vi "读取型号检测项.vi"(0 "产品型号路径":path, 5 "产品型号":string="potteryTemplete", 7 "树形List":refnum<vi>, 11 "error in (no error)":errorcluster caption="错误输入（无错误）") -> (15 "error out":errorcluster caption="错误输出")   [LabVIEW 2017]
uses:
  <vilib>/Utility/file.llb/Read Delimited Spreadsheet (string).vi
panel:
  out "添加的数组":string[][](array[string])
  out "大小":i32
  out "缩进格式数":i32[](array[numeric])
  out "all rows":string[][](array[string]) caption="所有行"
  out "添加的路径 2":path
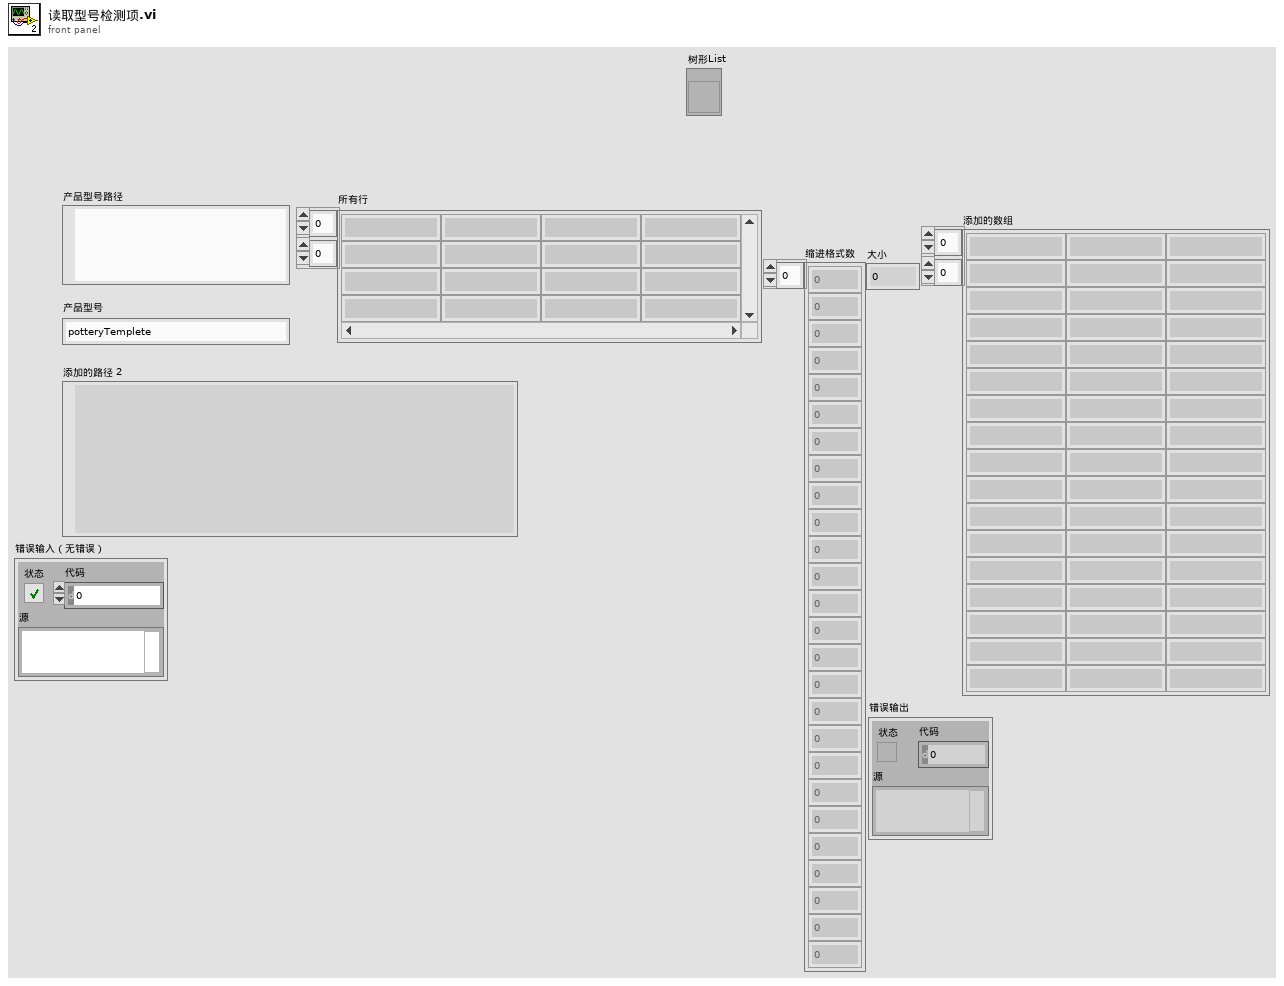
[diagram p1: front panel]
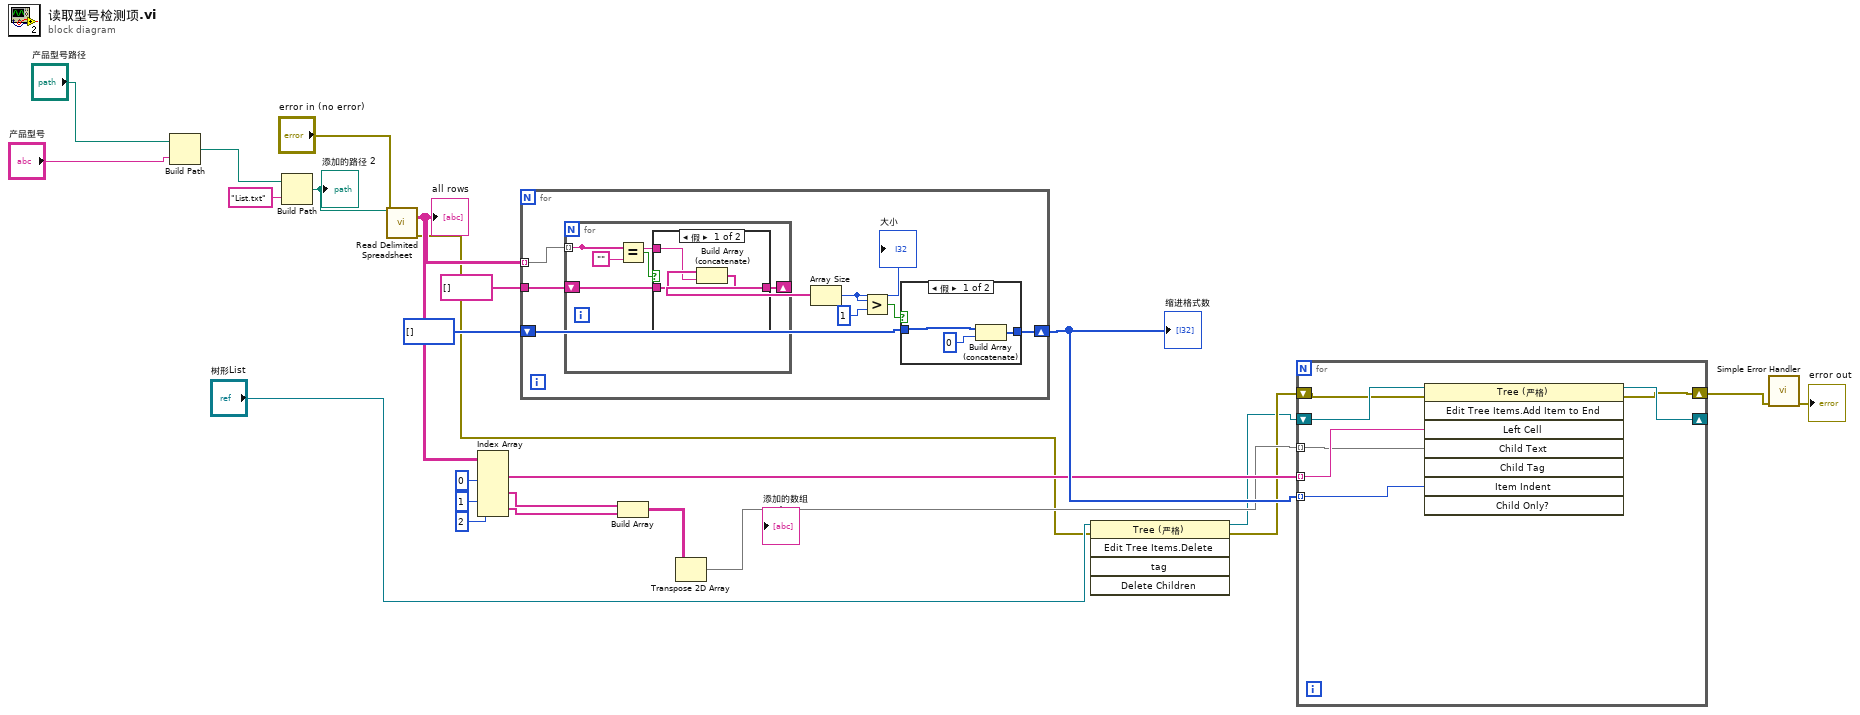
[diagram p0: block diagram]
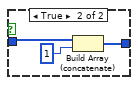
[diagram p3: hidden frame]
diagram:
  n1 = Build Path(base path="产品型号路径", name or relative path="产品型号") -> (appended path=w22:path)
  n2 = Build Path(base path=w22, name or relative path="List.txt" ("名称或相对路径")) -> (appended path=w20:path)
  "添加的路径 2" <- w20
  n3 = call-poly <vilib>:"Read Delimited Spreadsheet.vi"("file path (dialog if empty)"=w20, "error in (no error)"="error in (no error)") -> ("all rows"=w16:string[][], "error out"=w3:errorcluster)  [unwired: 8 in, 4 out]
  "all rows" <- w16
  n4 = Index Array(array=w16, index (col) #1=0 ("禁用的索引 (列)"), index (col) #2=1 ("索引 (列)"), index (col) #3=2 ("索引 (列)")) -> (element #1=w14:string[], element #2=w11:string[], element #3=w10:string[])  [unwired: 3 in]
  n5 = for {
    tunnel: w16 -> [w27] mode=indexing
    shift-right: [w28] -> w17
    shift-left: i32[] [] -> [w29]
    tunnel: string[] [] -> [w26]
    n6 = for {
      tunnel: w27 -> [w33] mode=indexing
      shift-right: [w34] -> w25
      shift-left: w26 -> [w35]
      n7 = Equal?(x=w33, y="") -> (x = y?=w36:bool)
      n8 = case shown="假" w36 {
        tunnel: w35 -> [w40 w41]
        tunnel: [w38 w41] -> w34
        tunnel: w33 -> [w39 _]
        frame False {
          n9 = Build Array (concatenate)(w40, w39) -> (w38:string[])
        }
        frame True {
        }
      }
    }
    n10 = Array Size(array=w25) -> (size(s)=w32:i32)
    "大小" <- w32
    n11 = Greater?(x=w32, y=1) -> (0:w30:bool)
    n12 = case shown="假" w30 {
      tunnel: w29 -> [w43 w47]
      tunnel: [w42 w45] -> w28
      frame False {
        n13 = Build Array (concatenate)(w43, 0 ("y")) -> (w42:i32[])
      }
      frame True {
        n14 = Build Array (concatenate)(w47, 1 ("y")) -> (w45:i32[])
      }
    }
  }
  "缩进格式数" <- w17
  n15 = Build Array(w11, w10) -> (w9:string[][])
  n16 = Transpose 2D Array(2D array=w9) -> (transposed array=w8:string[][])
  "添加的数组" <- w8
  n17 = invoke class="Tree (严格)" method="Edit Tree Items.Delete"(reference="树形List", error in=w3) -> (reference out=w1:refnum<vi>, error out=w2:errorcluster)  [unwired: 3 in, 3 out]
  n18 = for {
    tunnel: w17 -> [w50] mode=indexing
    tunnel: w14 -> [w52] mode=indexing
    tunnel: w8 -> [w51] mode=indexing
    shift-right: [w48] -> w7
    shift-left: w2 -> [w53]
    shift-right: [w49] -> _
    shift-left: w1 -> [w54]
    n19 = invoke class="Tree (严格)" method="Edit Tree Items.Add Item to End"(reference=w54, error in=w53, "Left Cell"=w52, "Child Text"=w51, "Item Indent"=w50) -> (reference out=w49:refnum<vi>, error out=w48:errorcluster)  [unwired: 3 in, 6 out]
  }
  n20 = call <vilib>:"Simple Error Handler.vi"("error in (no error)"=w7) -> ("error out"=→"error out":errorcluster)  [unwired: 4 in, 4 out]
